vi "GetNumLeds.vi"(8 "error in (no error)":errorcluster, 10 "Chain":i32, 11 "ControlState":T1 {"ChainMask" format="0x%02x"}) -> (0 "error out":errorcluster, 2 "NumLeds":i32, 3 "ControlState 2":T1 {"ChainMask" format="0x%02x"})   [LabVIEW 2023, in "ArduinoSerialBling.lvlib"]
uses:
  ArduinoSerialBling.lvlib
  ControlState.ctl
  ChainState.ctl
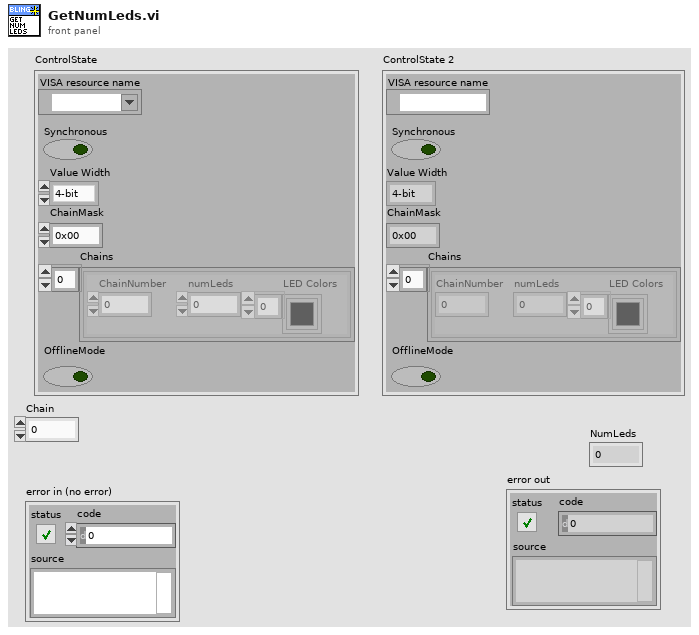
[diagram p1: front panel]
types:
  T1 = typedef "ArduinoSerialBling.lvlib/ControlState.ctl" = cluster{"VISA resource name":refnum<visa-resource-name>, "Synchronous":bool, "Value Width":enum16{"4-bit", "8-bit"}, "ChainMask":u8, "Chains":T2[], "OfflineMode":bool}
  T2 = typedef "ArduinoSerialBling.lvlib/ChainState.ctl" = cluster{"ChainNumber":u8, "numLeds":u8, "LED Colors":u32[]}
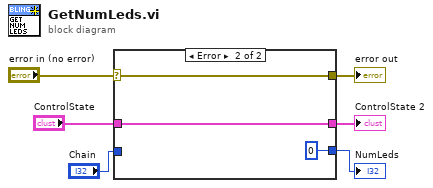
[diagram p0: block diagram]
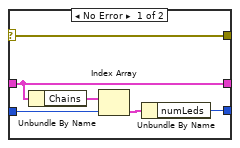
[diagram p2: hidden frame]
diagram:
  n1 = case shown="Error" "error in (no error)" {
    selector: "error in (no error)" -> [w12 w15]
    tunnel: [w12 w15] -> w5
    tunnel: "ControlState" -> [w11 w14]
    tunnel: [w11 w14] -> w3
    tunnel: "Chain" -> [w9 _]
    tunnel: [w7 u8 0 ("numLeds")] -> w1
    frame No Error {
      n2 = Unbundle By Name(w11) -> ("Chains"=w10:T2[])
      n3 = Index Array(array=w10, index=w9) -> (element=w8:T2)
      n4 = Unbundle By Name(w8) -> ("numLeds"=w7:u8)
    }
    frame Error {
    }
  }
  "ControlState 2" <- w3
  "error out" <- w5
  "NumLeds" <- w1
